vi "Ramp Up or Down (2D).vi"(0 "Array":dbl[][](array[numeric]), 2 "Down at end":bool, 7 "Sampling rate (Hz)":dbl, 9 "Ramp (ms)":dbl=5.0, 11 "Ramp up?":bool=TRUE, 12 "Start (0)":dbl, 13 "End (1)":dbl=1.0) -> (4 "Ramped array":dbl[][](array[numeric]), 8 "Ramp length":u32)   [LabVIEW 2020]
uses:
  PXI DAQ VIs/Utility VIs/Array Dimensions (2D).vi
  <vilib>/Analysis/NI_AALBase.lvlib
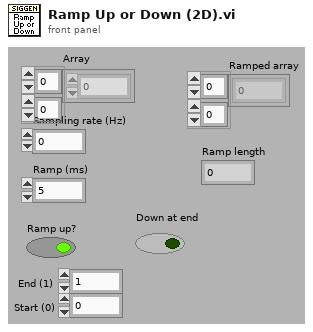
[diagram p1: front panel]
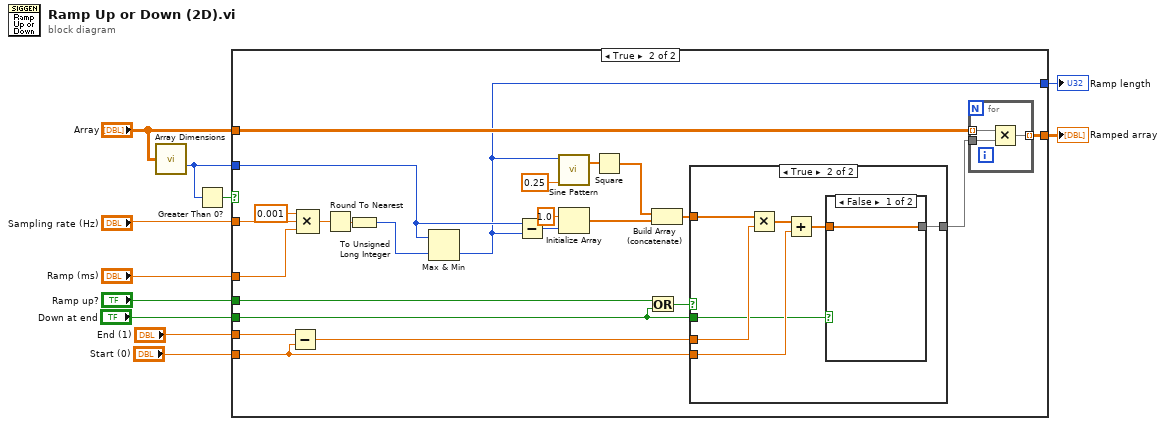
[diagram p0: block diagram]
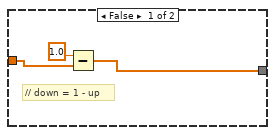
[diagram p3: hidden frame]
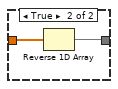
[diagram p4: hidden frame]
diagram:
  n1 = call-poly "Array Dimensions.vi"("2D Array"="Array") -> ("# columns"=w1:i32)  [unwired: 13 in, 1 out]
  n2 = Greater Than 0?(x=w1) -> (x > 0?=w8:bool)
  n3 = case shown="True" w8 {
    tunnel: "Ramp up?" -> [_ w15]
    tunnel: "Sampling rate (Hz)" -> [_ w30]
    tunnel: "Ramp (ms)" -> [_ w27]
    tunnel: w1 -> [_ w24]
    tunnel: "Array" -> [w12 w22]
    tunnel: [w12 w20] -> w6
    tunnel: "Start (0)" -> [_ w18]
    tunnel: "End (1)" -> [_ w19]
    tunnel: "Down at end" -> [_ w14]
    tunnel: [_ w13] -> w2
    frame False {
    }
    frame True {
      n4 = Subtract(x=w19, y=w18) -> (x-y=w17:dbl)
      n5 = Compound Arithmetic op=MULTIPLY(0.001 ("value"), w30, w27) -> (w31:dbl)
      n6 = Round To Nearest(number=w31) -> (nearest integer value=w36:dbl)
      n7 = To Unsigned Long Integer(number=w36) -> (unsigned 32bit integer=w23:u32)
      n8 = Max & Min(x=w24, y=w23) -> (min(x,y)=w13:u32)  [unwired: 1 out]
      n9 = Subtract(x=w24, y=w13) -> (x-y=w35:u32)
      n10 = call <vilib>:"Sine Pattern.vi"("cycles"=0.25, "samples"=w13) -> ("Sinusoidal Pattern"=w26:dbl[])  [unwired: 2 in, 1 out]
      n11 = Initialize Array(1.0 ("element"), w35) -> (w33:dbl[])
      n12 = Square(x=w26) -> (x^2=w25:dbl[])
      n13 = Or(x=w15, y=w14) -> (x .or. y?=w16:bool)
      n14 = Build Array (concatenate)(w25, w33) -> (w32:dbl[])
      n15 = case shown="True" w16 {
        tunnel: w32 -> [w41 w49]
        tunnel: [w40 w44] -> w21
        tunnel: w18 -> [_ w48]
        tunnel: w17 -> [_ w46]
        tunnel: w14 -> [_ w43]
        frame False {
          # "// down = 1 - up"
          n16 = Subtract(x=1.0, y=w41) -> (x-y=w40:dbl[])
        }
        frame True {
          n17 = Multiply(x=w49, y=w46) -> (x*y=w47:dbl[])
          n18 = Add(x=w47, y=w48) -> (x+y=w45:dbl[])
          n19 = case shown="False" w43 {
            tunnel: w45 -> [w50 w52]
            tunnel: [w50 w51] -> w44
            frame False {
            }
            frame True {
              n20 = Reverse 1D Array(array=w52) -> (reversed array=w51:dbl[])
            }
          }
        }
      }
      n21 = for {
        tunnel: w22 -> [w39] mode=indexing
        tunnel: w21 -> [w38]
        tunnel: [w37] -> w20 mode=indexing
        n22 = Multiply(x=w39, y=w38) -> (x*y=w37:dbl[])
      }
    }
  }
  "Ramped array" <- w6
  "Ramp length" <- w2
